vi "Meas Proc QWTB Fix Result Table Selection.vi"(7 "param table ref":refnum<vi>, 8 "error in":errorcluster) -> (0 "error out":errorcluster)   [LabVIEW 2018]
doc: "Detects position of the curcor in the table and sets selection to whole row accordingly."
uses:
  <vilib>/Utility/miscctls.llb/LVRowAndColumnTypeDef.ctl
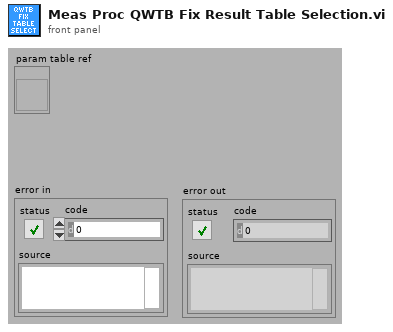
[diagram p1: front panel]
types:
  T1 = typedef "LVRowAndColumnTypeDef.ctl" = cluster{"Row":i32, "Column":i32}
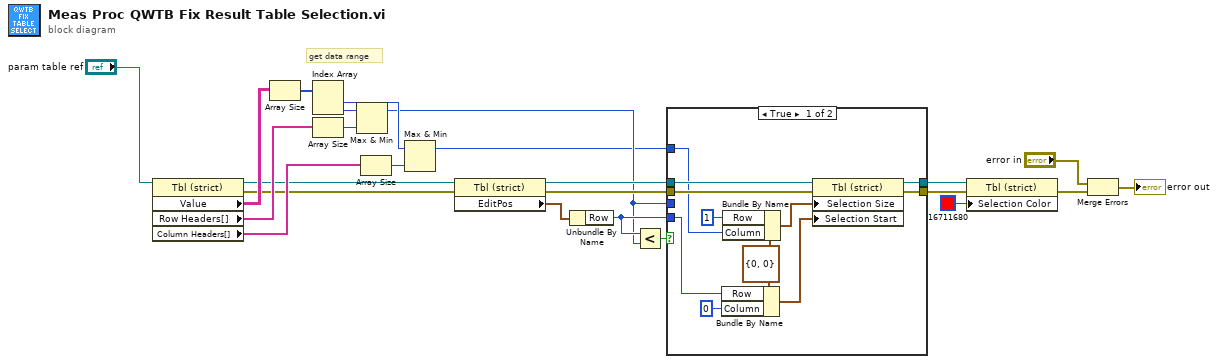
[diagram p0: block diagram]
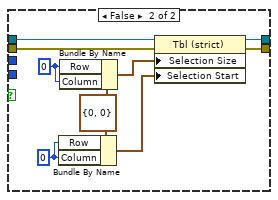
[diagram p2: hidden frame]
diagram:
  # "get data range"
  n1 = property class="Tbl (strict)"(reference="param table ref") -> (reference out=w13:refnum<vi>, error out=w10:errorcluster, "Value"=w22:string[][], "Row Headers[]"=w19:string[], "Column Headers[]"=w15:string[])  [unwired: 1 in]
  n2 = Array Size(array=w22) -> (size(s)=w21:i32[])
  n3 = Index Array(array=w21) -> (element #1=w14:i32, element #2=w20:i32)  [unwired: 2 in]
  n4 = Array Size(array=w19) -> (size(s)=w18:i32)
  n5 = Max & Min(x=w20, y=w18) -> (max(x,y)=w6:i32)  [unwired: 1 out]
  n6 = Array Size(array=w15) -> (size(s)=w16:i32)
  n7 = Max & Min(x=w14, y=w16) -> (max(x,y)=w5:i32)  [unwired: 1 out]
  n8 = property class="Tbl (strict)"(reference=w13, error in=w10) -> (reference out=w8:refnum<vi>, error out=w9:errorcluster, "EditPos"=w12:T1)
  n9 = Unbundle By Name(w12) -> ("Row"=w7:i32)
  n10 = Less?(x=w7, y=w6) -> (x < y?=w11:bool)
  n11 = case shown="True" w11 {
    tunnel: w9 -> [w35 w44]
    tunnel: w8 -> [w34 w43]
    tunnel: w7 -> [w25 _]
    tunnel: w6 -> [_ _]
    tunnel: w5 -> [w31 _]
    tunnel: [w27 w39] -> w4
    tunnel: [w26 w38] -> w3
    frame True {
      w30 = T1 {"Row"=0, "Column"=0} ("Selection Size")
      n12 = Bundle By Name(cluster=w30, "Row"=w25, "Column"=0) -> (w29:T1)
      n13 = Bundle By Name(cluster=w30, "Row"=1, "Column"=w31) -> (w33:T1)
      n14 = property class="Tbl (strict)"(reference=w34, error in=w35, "Selection Size"=w33, "Selection Start"=w29) -> (reference out=w26:refnum<vi>, error out=w27:errorcluster)
    }
    frame False {
      w36 = 0 ("Column")
      w37 = 0 ("Row")
      w41 = T1 {"Row"=0, "Column"=0} ("Selection Size")
      n15 = Bundle By Name(cluster=w41, "Row"=w36, "Column"=w36) -> (w40:T1)
      n16 = Bundle By Name(cluster=w41, "Row"=w37, "Column"=w37) -> (w42:T1)
      n17 = property class="Tbl (strict)"(reference=w43, error in=w44, "Selection Size"=w42, "Selection Start"=w40) -> (reference out=w38:refnum<vi>, error out=w39:errorcluster)
    }
  }
  n18 = property class="Tbl (strict)"(reference=w3, error in=w4, "Selection Color"=u32 16711680) -> (error out=w1:errorcluster)  [unwired: 1 out]
  n19 = Merge Errors("error in", w1) -> (→"error out":errorcluster)
